vi "导轨控制全局.vi"() -> ()   [LabVIEW 2015]
panel:
  in  "预置位位置":dbl
  in  "预置位巡检计数":dbl
  out "是否开始启用验证队列":bool
  in  "开始预置位巡检":bool
  in  "预置位状态":string
  in  "上下巡检状态":string
  in  "开始上下巡检":bool
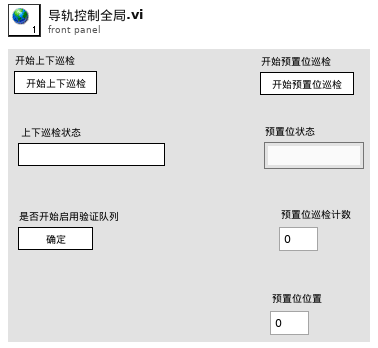
[diagram p1: front panel]
diagram:
